vi "FRCts20_Backend_Division_GET_reform.vi"(5 "Refnum in":T1, 7 "Division":T2, 8 "error in (no error)":errorcluster, 10 "Division":string, 11 "recordset data":variant[][](array[variant])) -> (0 "error out":errorcluster, 3 "data string":string)   [LabVIEW 2014]
uses:
  FRCts20_Backend_API/FRCts20_Backend_API_Division.ctl
  FRCts20_Backend_API/FRCts20_Backend_API_SW.ctl
  FRCts20_Backend_API/FRCts20_Backend_API_Status.ctl
  <vilib>/addons/database/Connection.llb/Conn ObjectReference.ctl
  FRCts20_Backend_DBCluster_Division_GET.ctl
  <vilib>/addons/database/_DB Variant To Data/Database Variant To Data.xnode
  FRCts20_Backend_Engine.lvlib
  FRCts20_Backend_API/FRCts20_Backend_API.lvlib
  <vilib>/addons/database/NI_Database_API.lvlib
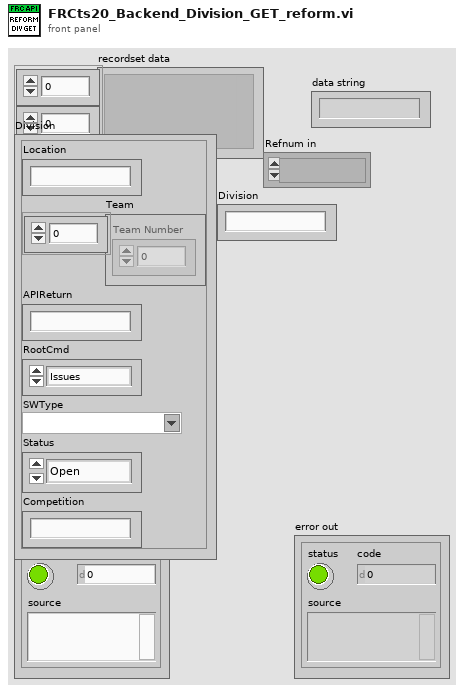
[diagram p1: front panel]
types:
  T1 = typedef "NI_Database_API.lvlib/Conn ObjectReference.ctl" = refnum<k1>
  T2 = typedef "FRCts20_Backend_API.lvlib/FRCts20_Backend_API_Division.ctl" = cluster{"Location":string, "Team":u32[], "APIReturn":string, "RootCmd":enum16{"Issues", "Software", "All"}, "SWType":T3, "Status":T4, "Competition":string}
  T3 = typedef "FRCts20_Backend_API.lvlib/FRCts20_Backend_API_SW.ctl" = string
  T4 = typedef "FRCts20_Backend_API.lvlib/FRCts20_Backend_API_Status.ctl" = enum16{"Open", "In Work", "Closed"}
  T5 = typedef "FRCts20_Backend_DBCluster_Division_GET.ctl" = cluster{"TeamNumber":u32}
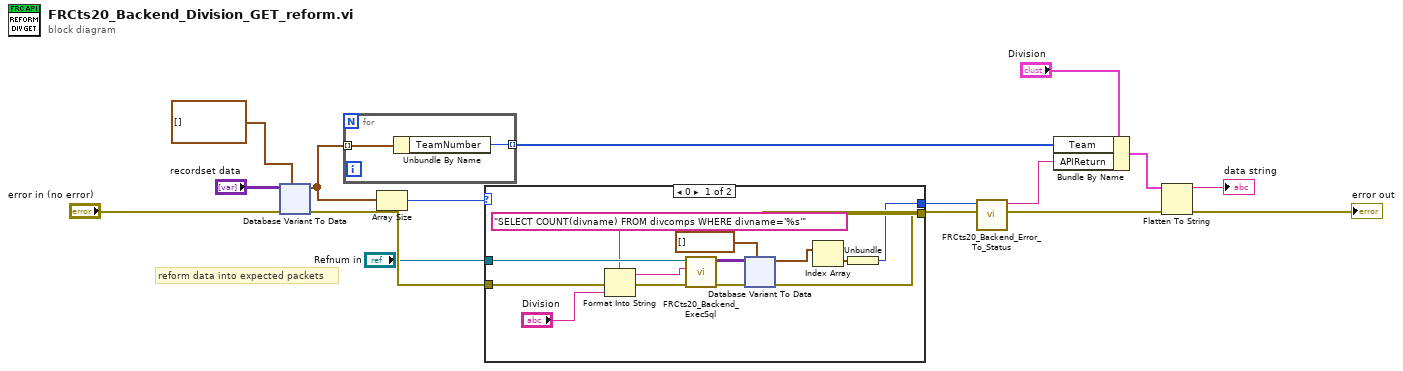
[diagram p0: block diagram]
diagram:
  # "reform data into expected packets"
  n1 = xnode "Database Variant To Data"("database variant"="recordset data", "error in (no error)"="error in (no error)", "type"=T5[] []) -> ("data"=w6:T5[], "error out"=w2:errorcluster)
  n2 = for {
    tunnel: [w18] -> w11 mode=indexing
    tunnel: w6 -> [w17] mode=indexing
    n3 = Unbundle By Name(w17) -> ("TeamNumber"=w18:u32)
  }
  n4 = Array Size(array=w6) -> (size(s)=w5:i32)
  n5 = case shown="0" w5 {
    selector: w5 -> [_ w74]
    tunnel: [w20 w74] -> w4
    tunnel: [w19 w73] -> w3
    tunnel: w2 -> [w26 w73]
    tunnel: "Refnum in" -> [w31 _]
    frame 0 {
      n6 = Format Into String(format string="SELECT COUNT(divname) FROM divcomps WHERE divname='%s'", error in=w26, "Division") -> (resulting string=w28:string, error out=w27:errorcluster)  [unwired: 1 in]
      n7 = call "FRCts20_Backend_ExecSql.vi"("error in (no error)"=w27, "format string"=w28, "Refnum in"=w31) -> ("error out"=w29:errorcluster, "recordset data"=w30:variant[][])  [unwired: 6 in, 1 out]
      n8 = xnode "Database Variant To Data"("database variant"=w30, "error in"=w29, "type"=cluster{u64}[] []) -> ("data"=w22:cluster{u64}[], "error out"=w19:errorcluster)
      n9 = Index Array(array=w22) -> (element=w21:cluster{u64})  [unwired: 1 in]
      n10 = Unbundle(w21) -> (w20:u64)
    }
    frame 1, Default {
    }
  }
  n11 = call "FRCts20_Backend_Error_To_Status.vi"("error in (no error)"=w3, "rows affected"=w4) -> ("error out"=w12:errorcluster, "String"=w13:string)  [unwired: 8 in]
  n12 = Bundle By Name(cluster="Division", "Team"=w11, "APIReturn"=w13) -> (w8:T2)
  n13 = Flatten To String(anything=w8, error in (no error)=w12) -> (data string=→"data string":string, error out=→"error out":errorcluster)  [unwired: 2 in, 1 out]
